vi "Get Point Iterator.vi"(0 "eye scan in":refnum<class "niHighSpeedSerial N Point Eye Scan v1 Host.lvclass">, 11 "error in":errorcluster) -> (4 "eye scan out":refnum<class "niHighSpeedSerial N Point Eye Scan v1 Host.lvclass">, 6 "eye scan point iterator":refnum<class "niHighSpeedSerial Eye Scan Point Iterator v1 Host.lvclass">, 15 "error out":errorcluster)   [LabVIEW 2014, in "niHighSpeedSerial N Point Eye Scan v1 Host.lvclass"]
doc: "Returns the Point Iterator.\n\n<B>Input Parameters</B>\n\n<B>eye scan in</B> Takes in a reference to your session from the previous VI.\n\n<B>error in</B> describes error conditions that occur before this node runs. This input provides standard 'error in' functionality.\n\n<B>Output Parameters</B>\n\n<B>eye scan out</B> passes a reference to your session to the next VI.\n\n<B>eye scan point iterator</B> is the incoming wire for the Eye Scan Point Iterator class object\n\n<B>error out</B> contains error information. This output provides standard 'error out' functionality."
uses:
  <instrlib>/niHighSpeedSerial/Eye Scan/v1/Host/Impl/N Point Eye Scan/niHighSpeedSerial N Point Eye Scan v1 Host.lvclass
  <instrlib>/niHighSpeedSerial/Eye Scan/v1/Host/Impl/Eye Scan Point Iterator/niHighSpeedSerial Eye Scan Point Iterator v1 Host.lvclass
  <instrlib>/niHighSpeedSerial/Eye Scan/v1/Host/Impl/N Point Eye Scan/niHighSpeedSerial N Point Eye Scan v1 Host.lvclass/niHighSpeedSerial N Point Eye Scan v1 Host.ctl
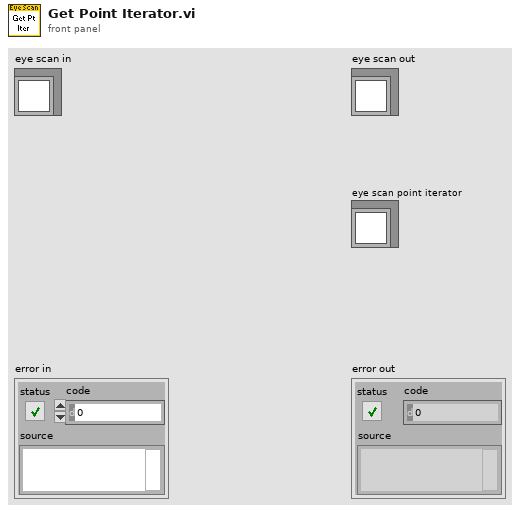
[diagram p1: front panel]
types:
  T1 = typedef "N Point Eye Scan v1 Host.lvclass/Private Data.ctl" = cluster{"array of points to measure":T2[], "n point eye scan point iterator":refnum<class "niHighSpeedSerial N Point Eye Scan Point Iterator v1 Host.lvclass">}
  T2 = typedef "niHighSpeedSerial Eye Scan Common v1 Host.lvlib/Point Offsets.ctl" = cluster{"horizontal offset":i16, "vertical offset":i8}
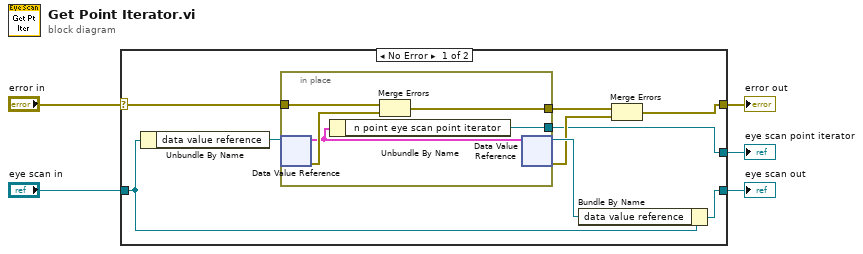
[diagram p0: block diagram]
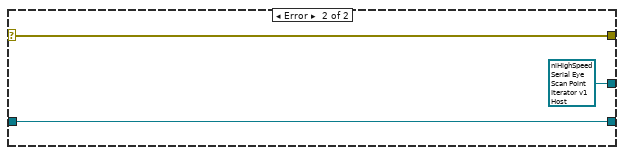
[diagram p2: hidden frame]
diagram:
  n1 = case shown="No Error" "error in" {
    selector: "error in" -> [w10 w22]
    tunnel: [w8 w22] -> w4
    tunnel: [w11 w21] -> w3
    tunnel: "eye scan in" -> [w13 w21]
    tunnel: [w6 refnum<class "niHighSpeedSerial Eye Scan Point Iterator v1 Host.lvclass"> refnum ("Point Iterator")] -> w1
    frame No Error {
      n2 = Unbundle By Name(w13) -> ("data value reference"=w14:refnum<data-value>)
      n3 = in-place {
        in-place-border: w10 -> [w18]
        in-place-border: [w16] -> w7
        in-place-border: [w19] -> w6
        n4 = in-place-dvr #1(w14) -> (w15:T1, w17:errorcluster)
        n5 = Unbundle By Name(w15) -> ("n point eye scan point iterator"=w19:refnum<class "niHighSpeedSerial N Point Eye Scan Point Iterator v1 Host.lvclass">)
        n6 = Merge Errors(w18, w17) -> (w16:errorcluster)
        n7 = in-place-dvr #1(w15) -> (w12:refnum<data-value>, w9:errorcluster)
      }
      n8 = Bundle By Name(cluster=w13, "data value reference"=w12) -> (w11:refnum<class "niHighSpeedSerial N Point Eye Scan v1 Host.lvclass">)
      n9 = Merge Errors(w7, w9) -> (w8:errorcluster)
    }
    frame Error {
    }
  }
  "error out" <- w4
  "eye scan out" <- w3
  "eye scan point iterator" <- w1
